vi "New PDF.vi"(0 "PDF Path":path, 1 "Unit (default = mm)":T3=enum."mm", 2 "Overwrite?":bool=TRUE, 3 "Captions":T4={"Figure"={"Caption"="Figure", "Separator"="  ", "Position"=enum."Below"}, "Table"={"Caption"="Table", "Separator"="  ", "Position"=enum."Above"}, "Font"={"Name"="", "Size"=-1.0, "Color"=0, "Style"={"Bold"=FALSE, "Italic"=FALSE, "Underline"=FALSE, "Strikeout"=FALSE}, "Type"={"Type&direction"=enum."Select", "Embedded"=FALSE, "Encoding"=""}}}, 5 "Default Font":T6={"Name"="Arial", "Size"=12.0, "Color"=0, "Style"={"Bold"=FALSE, "Italic"=FALSE, "Underline"=FALSE, "Strikeout"=FALSE}, "Type"={"Type&direction"=enum."ASCII", "Embedded"=FALSE, "Encoding"=""}}, 7 "At the opening":T1={"Page"=0, "Show Bookmarks"=TRUE} {"Page" items=["Single Page - Fit Page"=1, "Single Page - Fit Width"=0]}, 9 "Default Paragraph":T11={" Aligment"=enum."JUSTIFY", "Line spacing"=enum."1.0"}, 11 "error in (no error)":errorcluster, 12 "Page Setup":T15={"Page Size"=1, "Orientation"=enum."Portrait", "Custom Size"={"Width"=216.0, "Height"=279.0}, "Margins"={"Left"=25.0, "Right"=25.0, "Top"=25.0, "Bottom"=25.0}} {"Page Size" items=["Custom", "LETTER", "NOTE", "LEGAL", "TABLOID", "EXECUTIVE", "POSTCARD", "A0", "A1", "A2", "A3", "A4", "A5", "A6", "A7", "A8", "A9", "A10", "B0", "B1", "B2", "B3", "B4", "B5", "B6", "B7", "B8", "B9", "B10", "ARCH_E", "ARCH_D", "ARCH_C", "ARCH_B", "ARCH_A", "FLSA", "FLSE", "HALFLETTER", "_11X17", "ID_1", "ID_2", "ID_3", "LEDGER", "CROWN_QUARTO", "LARGE_CROWN_QUARTO", "DEMY_QUARTO", "ROYAL_QUARTO", "CROWN_OCTAVO", "LARGE_CROWN_OCTAVO", "DEMY_OCTAVO", "ROYAL_OCTAVO", "SMALL_PAPERBACK", "PENGUIN_SMALL_PAPERBACK", "PENGUIN_LARGE_PAPERBACK"]}, 13 "PDF Details":T14={"Title"="", "Author"="", "Subject"="", "Keywords"="", "Creator"="Exaprom PDF"}, 14 "Permissions":T2={"User Password"="", "Owner Password"="", "Printing"=enum."Allow Printing", "Allow Modify Contents"=TRUE, "Allow Copy"=TRUE, "Allow Modify Annotations"=TRUE, "Allow Fill In "=TRUE, "Allow Screen Readers"=TRUE, "Allow Assembly"=TRUE}) -> (4 "PDF Report":refnum<class "PDF Report Class.lvclass">, 15 "error out":errorcluster)   [LabVIEW 2019]
doc: "Set the default values:\n1) Captions;\n2) Overwrite?;\n3) File or Directory path;\n4) Page Setup;\n5) PDF Details;\n6) Unit (default mm);\n7) Default font;\n8) Default Paragraph;\n\n<B>1) Captions </B>\nCaptions for tables and figures.\n\n<B>2) Overwrite?</B>\n\n<B>3) File or Directory path</B>\n\n<B>4)Page Setup</B>\n- Page size\n- Orientation\n- Margins\n- Custom layout (if Page size = custom)\n\n<B>5) PDF Details</B> \n- Title\n- Subject\n- Keyword\n- Author\n- Creator\n\n<B>6) Unit (default mm)</B>\nmm or in: unit used in all the report except when the unit \"point\" is specified\n\n<B>7) Default font</B>\n\nDefault font for all the report (fonts available in C:\\Windows\\Fonts).\n\n<B>8) Default Paragraph</B>\n- Alignment\n- Line Spacing\n\n<B>FRANÇAIS </B>\n\nCréation du rapport avec les paramètres par défauts:\n\n1) Légendes \"Captions\";\n2) Écrire par dessus un fichier existant \"Overwrite?\"\n3) Répertoire ou le nom du fichier \"File or Directory path\";\n4) Format des pages \"Page Setup\";\n5) Détails du fichier PDF \"PDF Details\";\n6) Unité par défaut \"Unit (default mm)\";\n7) Police de caractères par défaut \"Default font\";\n8) Interligne et l'alignement par défaut \"Default Paragraph\";\n\n<B>1) Légendes \"Captions\"</B>\nLes intitulés génériques pour les légendes (Captions) des figures et tableaux.\n\n<B>2) Écrire par dessus un fichier existant \"Overwrite?\"</B>\n\n<B>3) Répertoire ou le nom du fichier \"File or Directory path\";</B>\nLe répertoire ou le nom du fichier (chemin complet) à utiliser.\n\n<B>4) Format des pages \"Page Setup\" </B>\nFormat des pages incluant:\n- l'orientation (portrait ou paysage)\n- les marges;\n- la taille exacte si c'est un format personnalisé.\n\n<B>5) Détails du fichier PDF \"PDF Details\"</B> (métadonnées)\n- titre\n- sujet\n- mots-clés\n- auteur\n- créateur\n\n<B>6) Unité par défaut \"Unit (default mm)\"</B>\nmm or in: l'unité utilise dans l'ensemble du rapport excepté ou l'unité \"point\" spécifiée.\n\n<B>7) Police de caractères par défaut \"Default font\"</B>\n\nPolice de caractères par défaut du rapport (police disponible dans C:\\Windows\\Fonts).\n\n<B>8) Interligne et l'alignement par défaut \"Default Paragraph\"</B>\n- alignement;\n- interligne (1.0, 1.5 et 2.0)\n\nVersion 2.0\nDeveloped by Jean-Marc Simard\nCopyright © 2012, Exaprom Inc.\nAll rights reserved.\nLicense: BSD\n\nWith iTextSharp 4.1.6 (http://itextsharp.sourceforge.net)\nunder Mozilla Public License Version 1.1\n(http://www.mozilla.org/MPL/MPL-1.1.html)"
uses:
  <userlib>/Exaprom PDF/Controls/Page Controls/Page setup.ctl
  <userlib>/Exaprom PDF/Controls/Page Controls/Page size.ctl
  <userlib>/Exaprom PDF/Controls/Page Controls/Page Orientation.ctl
  <userlib>/Exaprom PDF/Controls/Page Controls/Page Layout Custom.ctl
  <userlib>/Exaprom PDF/Controls/Page Controls/Page margins.ctl
  <userlib>/Exaprom PDF/LV Class/PDF Report Class/PDF Report Class.lvclass
  <userlib>/Exaprom PDF/Controls/Initialization Controls/PDF Details.ctl
  <userlib>/Exaprom PDF/Controls/Font Controls/Font complete cluster.ctl
  <userlib>/Exaprom PDF/Controls/Font Controls/Font size.ctl
  <userlib>/Exaprom PDF/Controls/Font Controls/Font color.ctl
  <userlib>/Exaprom PDF/Controls/Font Controls/Type and encoding.ctl
  <userlib>/Exaprom PDF/Controls/Text Controls/Unicode/Type and run direction.ctl
  <userlib>/Exaprom PDF/Controls/Initialization Controls/Defaut Paragraphe and Line Spacing.ctl
  <userlib>/Exaprom PDF/Controls/Text Controls/Texte alignement.ctl
  <userlib>/Exaprom PDF/Controls/Text Controls/Line spacing.ctl
  <userlib>/Exaprom PDF/Controls/Initialization Controls/Captions.ctl
  <userlib>/Exaprom PDF/Controls/Initialization Controls/Image or Table Caption.ctl
  <userlib>/Exaprom PDF/Controls/Initialization Controls/Unit.ctl
  <userlib>/Exaprom PDF/Controls/Initialization Controls/File Permission Parameters.ctl
  <userlib>/Exaprom PDF/Controls/Initialization Controls/At the opening.ctl
  <userlib>/Exaprom PDF/Controls/General Controls/Create, open or close.ctl
  <userlib>/Exaprom PDF/LV Class/Fonts Class/Font Class.lvclass
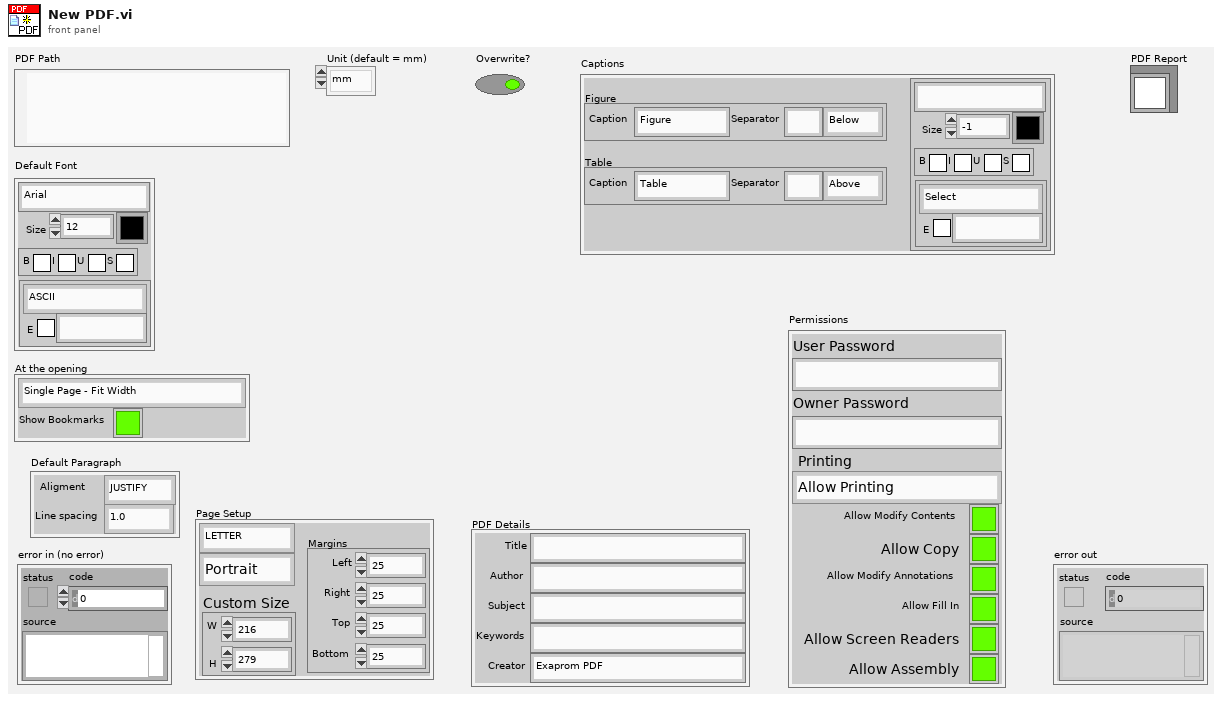
[diagram p1: front panel]
types:
  T1 = typedef "At the opening.ctl" = cluster{"Page":u16, "Show Bookmarks":bool}
  T2 = typedef "File Permission Parameters.ctl" = cluster{"User Password":string, "Owner Password":string, "Printing":enum16{"Allow Printing", "Allow Degraded Printing", "Don't Allow Printing"}, "Allow Modify Contents":bool, "Allow Copy":bool, "Allow Modify Annotations":bool, "Allow Fill In ":bool, "Allow Screen Readers":bool, "Allow Assembly":bool}
  T3 = typedef "Unit.ctl" = enum16{"inch", "mm"}
  T4 = typedef "Captions.ctl" = cluster{"Figure":T5, "Table":T5, "Font":T6}
  T5 = typedef "Image or Table Caption.ctl" = cluster{"Caption":string, "Separator":string, "Position":enum16{"Above", "Below"}}
  T6 = typedef "Font complete cluster.ctl" = cluster{"Name":string, "Size":T7, "Color":T8, "Style":cluster{"Bold":bool, "Italic":bool, "Underline":bool, "Strikeout":bool}, "Type":T9}
  T7 = typedef "Font size.ctl" = sgl
  T8 = typedef "Font color.ctl" = u32
  T9 = typedef "Type and encoding.ctl" = cluster{"Type&direction":T10, "Embedded":bool, "Encoding":string}
  T10 = typedef "Type and run direction.ctl" = enum16{"Select", "ASCII", "UTF-16", "UTF-16 (default)", "UTF-16 (LTR)", "UTF-16 (RTL)"}
  T11 = typedef "Defaut Paragraphe and Line Spacing.ctl" = cluster{" Aligment":T12, "Line spacing":T13}
  T12 = typedef "Texte alignement.ctl" = enum16{"Select", "CENTER", "JUSTIFY", "LEFT", "RIGHT"}
  T13 = typedef "Line spacing.ctl" = enum16{"Select", "1.0", "1.5", "2.0"}
  T14 = typedef "PDF Details.ctl" = cluster{"Title":string, "Author":string, "Subject":string, "Keywords":string, "Creator":string}
  T15 = typedef "Page setup.ctl" = cluster{"Page Size":T16, "Orientation":T17, "Custom Size":T18, "Margins":T19}
  T16 = typedef "Page size.ctl" = i32
  T17 = typedef "Page Orientation.ctl" = enum16{"Portrait", "Landscape"}
  T18 = typedef "Page Layout Custom.ctl" = cluster{"Width":sgl, "Height":sgl}
  T19 = typedef "Page margins.ctl" = cluster{"Left":sgl, "Right":sgl, "Top":sgl, "Bottom":sgl}
  T20 = typedef "Create, open or close.ctl" = enum16{"Create", "Open", "Close"}
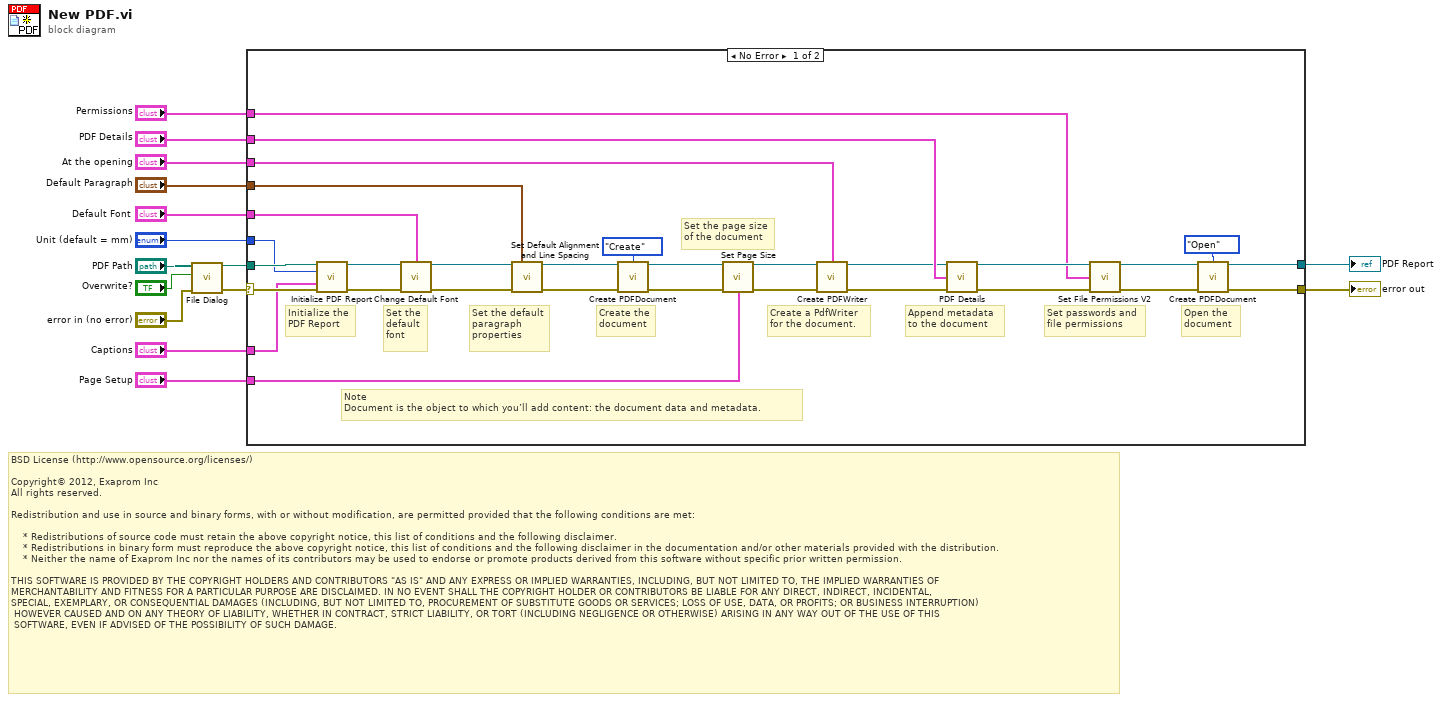
[diagram p0: block diagram]
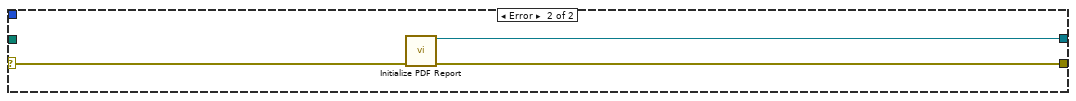
[diagram p2: hidden frame]
diagram:
  # "BSD License (http://www.opensource.org/licenses/)\n\nCopyright© 2012, Exaprom Inc\nAll rights reserved.\n\nRedistribution and use in source and binary forms, with or without modification, are permitted provided that the following conditions are met:\n\n    * Redistributions of source code must retain the above copyright notice, this list of conditions and the following disclaimer.\n    * Redistributions in binary form must reproduce the above copyright notice, this list of conditions and the following disclaimer in the documentation and/or other materials provided with the distribution.\n    * Neither the name of Exaprom Inc nor the names of its contributors may be used to endorse or promote products derived from this software without specific prior written permission.\n\nTHIS SOFTWARE IS PROVIDED BY THE COPYRIGHT HOLDERS AND CONTRIBUTORS \"AS IS\" AND ANY EXPRESS OR IMPLIED WARRANTIES, INCLUDING, BUT NOT LIMITED TO, THE IMPLIED WARRANTIES OF \nMERCHANTABILITY AND FITNESS FOR A PARTICULAR PURPOSE ARE DISCLAIMED. IN NO EVENT SHALL THE COPYRIGHT HOLDER OR CONTRIBUTORS BE LIABLE FOR ANY DIRECT, INDIRECT, INCIDENTAL,\nSPECIAL, EXEMPLARY, OR CONSEQUENTIAL DAMAGES (INCLUDING, BUT NOT LIMITED TO, PROCUREMENT OF SUBSTITUTE GOODS OR SERVICES; LOSS OF USE, DATA, OR PROFITS; OR BUSINESS INTERRUPTION)\n HOWEVER CAUSED AND ON ANY THEORY OF LIABILITY, WHETHER IN CONTRACT, STRICT LIABILITY, OR TORT (INCLUDING NEGLIGENCE OR OTHERWISE) ARISING IN ANY WAY OUT OF THE USE OF THIS\n SOFTWARE, EVEN IF ADVISED OF THE POSSIBILITY OF SUCH DAMAGE."
  n1 = call <userlib>:"File Dialog.vi"("error in (no error)"="error in (no error)", "Overwrite?"="Overwrite?", "Path In"="PDF Path") -> ("error out"=w9:errorcluster, "Path Out"=w11:path)  [unwired: 7 out]
  n2 = case shown="No Error" w9 {
    selector: w9 -> [w40 w47]
    tunnel: "Page Setup" -> [w45 _]
    tunnel: "PDF Details" -> [w44 _]
    tunnel: "Default Font" -> [w41 _]
    tunnel: "Default Paragraph" -> [w43 _]
    tunnel: w11 -> [w38 _]
    tunnel: [w20 w48] -> w8
    tunnel: "Captions" -> [w36 _]
    tunnel: "Unit (default = mm)" -> [w37 _]
    tunnel: [w19 w46] -> w4
    tunnel: "Permissions" -> [w33 _]
    tunnel: "At the opening" -> [w16 _]
    frame No Error {
      # "Create the\ndocument"
      # "Set passwords and\nfile permissions"
      # "Note\nDocument is the object to which you’ll add content: the document data and metadata."
      # "Open the\ndocument"
      # "Append metadata\nto the document"
      # "Create a PdfWriter \nfor the document."
      # "Set the page size\nof the document"
      # "Set the default\nparagraph \nproperties"
      # "Set the\ndefault \nfont"
      # "Initialize the \nPDF Report"
      n3 = call <userlib>:"Initialize PDF Report.vi"("PDF Path"=w38, "Unit (default = mm)"=w37, "Captions"=w36, "error in (no error)"=w40) -> ("PDF Report"=w39:refnum<class "PDF Report Class.lvclass">, "error out (no error)"=w42:errorcluster)  [unwired: 10 in]
      n4 = call <userlib>:"Change Default Font.vi"("PDF Report IN"=w39, "Font"=w41, "error in (no error)"=w42) -> ("PDF Report OUT"=w17:refnum<class "PDF Report Class.lvclass">, "error out"=w18:errorcluster)  [unwired: 11 in]
      n5 = call <userlib>:"Set Default Alignment and Line Spacing.vi"("PDF Report IN"=w17, "Default Paragraph"=w43, "error in (no error)"=w18) -> ("PDF Report IN"=w26:refnum<class "PDF Report Class.lvclass">, "error out"=w27:errorcluster)  [unwired: 11 out]
      n6 = call <userlib>:"Create PDFDocument.vi"("PDF Report IN"=w26, "Open or create"=Create,_open_or_close."Create", "error in (no error)"=w27) -> ("PDF Report OUT"=w25:refnum<class "PDF Report Class.lvclass">, "error out"=w28:errorcluster)  [unwired: 11 in]
      n7 = call <userlib>:"Set Page Size.vi"("PDF Report IN"=w25, "Page setup"=w45, "error in (no error)"=w28) -> ("PDF Report OUT"=w29:refnum<class "PDF Report Class.lvclass">, "error OUT"=w30:errorcluster)  [unwired: 11 out]
      n8 = call <userlib>:"Create PDFWriter.vi"("PDF Report IN"=w29, "At the opening"=w16, "error in (no error)"=w30) -> ("PDF Report OUT"=w31:refnum<class "PDF Report Class.lvclass">, "error out"=w32:errorcluster)  [unwired: 11 in]
      n9 = call <userlib>:"PDF Details.vi"("PDF Report IN"=w31, "PDF Details"=w44, "error in (no error)"=w32) -> ("PDF Report OUT"=w34:refnum<class "PDF Report Class.lvclass">, "error out"=w35:errorcluster)  [unwired: 11 in]
      n10 = call <userlib>:"Set File Permissions V2.vi"("PDF Report IN"=w34, "Permissions"=w33, "error in (no error)"=w35) -> ("PDF Report OUT"=w22:refnum<class "PDF Report Class.lvclass">, "error out"=w23:errorcluster)  [unwired: 11 out]
      n11 = call <userlib>:"Create PDFDocument.vi"("PDF Report IN"=w22, "Open or create"=Create,_open_or_close."Open", "error in (no error)"=w23) -> ("PDF Report OUT"=w19:refnum<class "PDF Report Class.lvclass">, "error out"=w20:errorcluster)  [unwired: 11 in]
    }
    frame Error {
      n12 = call <userlib>:"Initialize PDF Report.vi"("error in (no error)"=w47) -> ("PDF Report"=w46:refnum<class "PDF Report Class.lvclass">, "error out (no error)"=w48:errorcluster)  [unwired: 13 in]
    }
  }
  "error out" <- w8
  "PDF Report" <- w4
